vi "Phasor Compare Calibrations.vi"(9 "new Calibration Phasor":T1, 11 "old Calibration Phasor":T1) -> (3 "Calibration changed":bool)   [LabVIEW 2021, in "Phasor.lvlib"]
doc: "Compares two calibrations.\n\nIf m = NaN (interpreted as \"Use nearest valid calibration\", a standard comparison test will fail because NaN != NaN, hence the need for this VI to report whether any of the components is different."
uses:
  Calibration Phasor (m, phi).ctl
  Phasor.lvlib
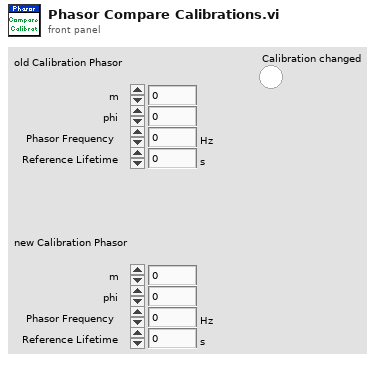
[diagram p1: front panel]
types:
  T1 = typedef "Phasor.lvlib/Calibration Phasor (m, phi).ctl" = cluster{"m":dbl, "phi":dbl, "Phasor Frequency":dbl[unit], "Reference Lifetime":dbl[unit]}
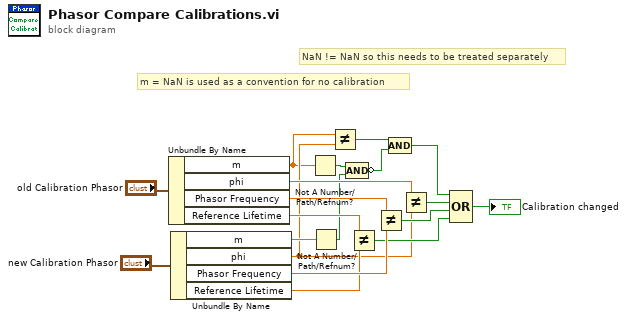
[diagram p0: block diagram]
diagram:
  # "NaN != NaN so this needs to be treated separately"
  # "m = NaN is used as a convention for no calibration"
  n1 = Unbundle By Name("old Calibration Phasor") -> ("m"=w7:dbl, "phi"=w17:dbl, "Phasor Frequency"=w16:dbl[unit], "Reference Lifetime"=w14:dbl[unit])
  n2 = Unbundle By Name("new Calibration Phasor") -> ("m"=w12:dbl, "phi"=w8:dbl, "Phasor Frequency"=w15:dbl[unit], "Reference Lifetime"=w13:dbl[unit])
  n3 = Not A Number/Path/Refnum?(number/path/refnum=w7) -> (NaN/Path/Refnum?=w6:bool)
  n4 = Not A Number/Path/Refnum?(number/path/refnum=w12) -> (NaN/Path/Refnum?=w5:bool)
  n5 = Not Equal?(x=w7, y=w8) -> (x != y?=w4:bool)
  n6 = Compound Arithmetic op=AND(w6, w5) -> (invert w3:bool)
  n7 = Not Equal?(x=w14, y=w13) -> (x != y?=w9:bool)
  n8 = Not Equal?(x=w16, y=w15) -> (x != y?=w10:bool)
  n9 = Compound Arithmetic op=AND(w4, w3) -> (w2:bool)
  n10 = Not Equal?(x=w17, y=w8) -> (x != y?=w11:bool)
  n11 = Compound Arithmetic op=OR(w2, w11, w10, w9) -> (→"Calibration changed":bool)
